vi "32-bit Main.vi"() -> ()   [LabVIEW 2017]
uses:
  <vilib>/express/express analysis/Spectral/Block/exnSpectralBlock spectral measurements peak poly.vi
  <vilib>/express/express analysis/Spectral/Block/exnSpectralBlock spectral measurements peak WFM.vi
  <vilib>/express/express analysis/Spectral/XNode/ExpressSpectralMeasurementsBlockNode.xnode
panel:
  out "Error 401007":errorcluster
  out "Waveform Chart 401007":dbl(graph)
  out "Unsigned Byte Array 401007":u8[](array[numeric])
  out "Little Endian":dbl
  in  "Big Endian":dbl
  out "303005":dbl
  out "Error 303005":errorcluster
  out "Error 303005.1":errorcluster
  out "303005.1":dbl
  out "303007":i64
  out "Error 303007":errorcluster
  out "Error 401007":errorcluster
  out "401007":dbl
  out "Error 401001":errorcluster
  out "401001":i64
  out "Error 301001":errorcluster
  out "301001":i64
  out "Error 001001":errorcluster
  out "001001":bool
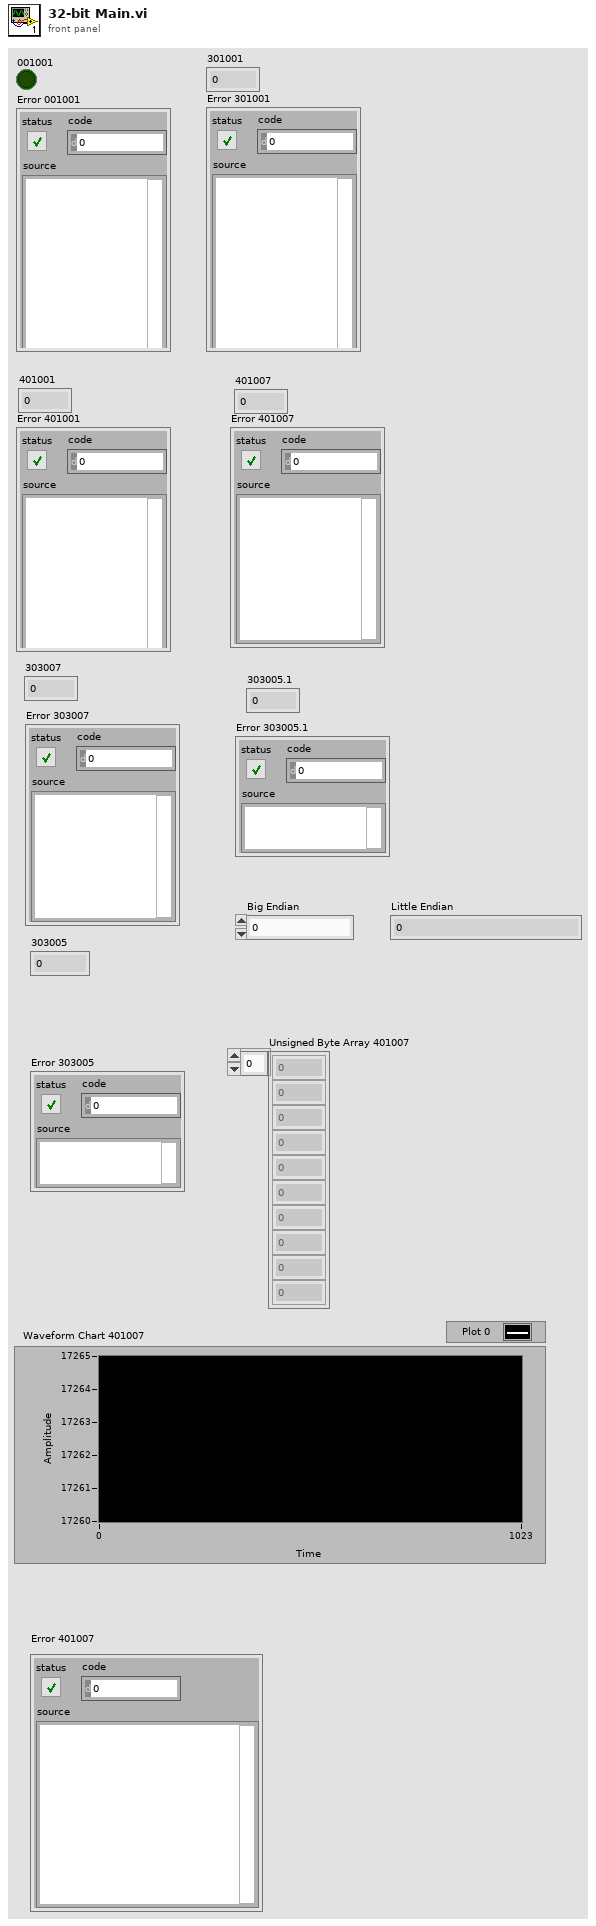
[diagram p1: front panel]
types:
  T1 = enum16{"big-endian, network order", "native, host order", "little-endian"}
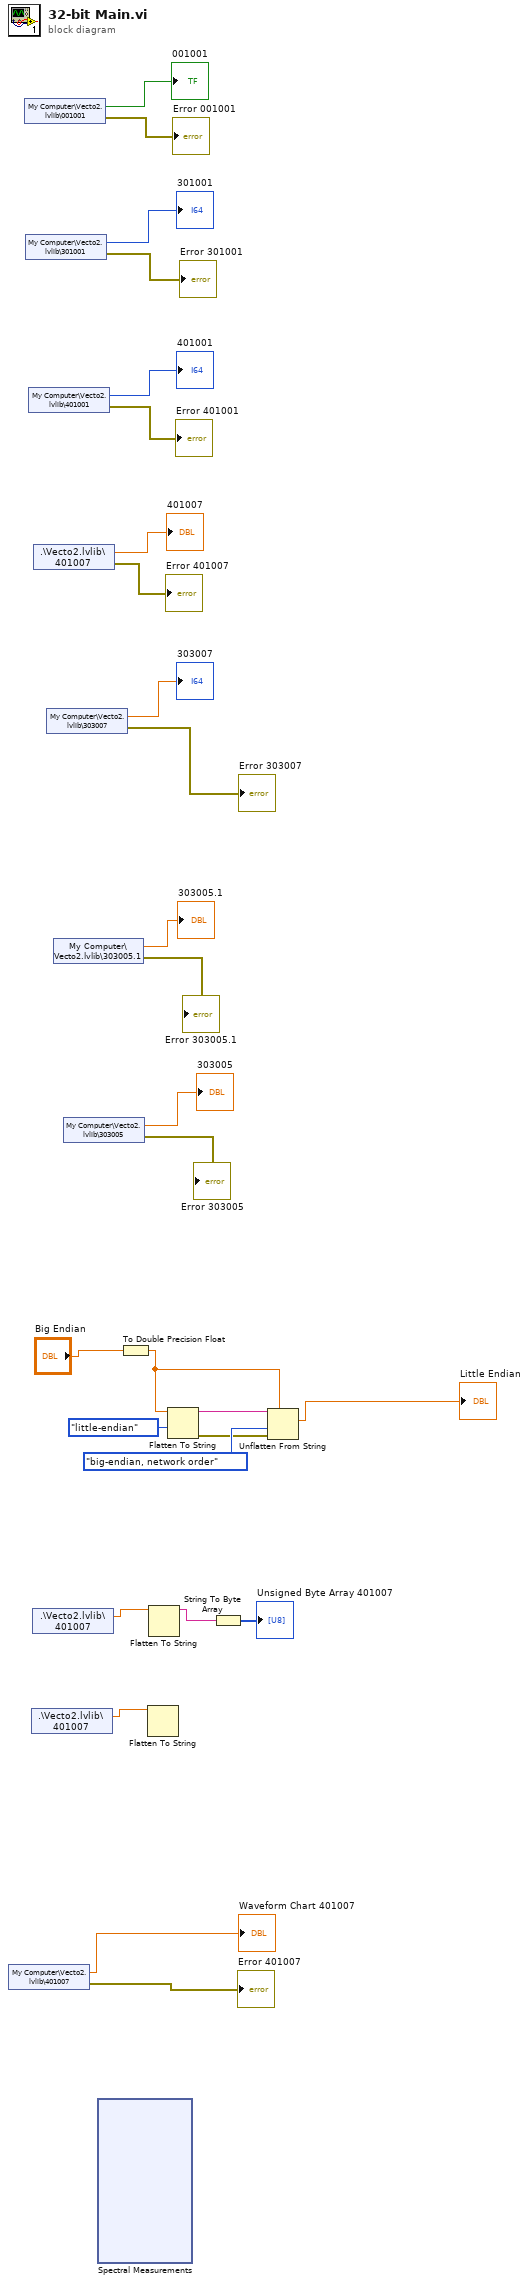
[diagram p0: block diagram]
diagram:
  n1 = shared-variable "My Computer\\Vecto2.lvlib\\401007"() -> (→"Waveform Chart 401007":dbl, error out=→"Error 401007":errorcluster)  [unwired: 1 in]
  n2 = shared-variable "My Computer\\Vecto2.lvlib\\001001"() -> (→"001001":bool, error out=→"Error 001001":errorcluster)  [unwired: 1 in]
  n3 = shared-variable "My Computer\\Vecto2.lvlib\\301001"() -> (→"301001":i64, error out=→"Error 301001":errorcluster)  [unwired: 1 in]
  n4 = shared-variable "My Computer\\Vecto2.lvlib\\401001"() -> (→"401001":i64, error out=→"Error 401001":errorcluster)  [unwired: 1 in]
  n5 = shared-variable ".\\Vecto2.lvlib\\401007"() -> (w2:dbl)  [unwired: 1 in, 1 out]
  n6 = shared-variable ".\\Vecto2.lvlib\\401007"() -> (w7:dbl)  [unwired: 1 in, 1 out]
  n7 = shared-variable ".\\Vecto2.lvlib\\401007"() -> (→"401007":dbl, error out=→"Error 401007":errorcluster)  [unwired: 1 in]
  n8 = shared-variable "My Computer\\Vecto2.lvlib\\303007"() -> (→"303007":sgl, error out=→"Error 303007":errorcluster)  [unwired: 1 in]
  n9 = shared-variable "My Computer\\Vecto2.lvlib\\303005.1"() -> (→"303005.1":dbl, error out=→"Error 303005.1":errorcluster)  [unwired: 1 in]
  n10 = shared-variable "My Computer\\Vecto2.lvlib\\303005"() -> (→"303005":dbl, error out=→"Error 303005":errorcluster)  [unwired: 1 in]
  n11 = xnode "Spectral Measurements"() -> ()  [unwired: 2 in, 3 out]
  n12 = To Double Precision Float(number="Big Endian") -> (double precision float=w9:dbl)
  n13 = Flatten To String(anything=w2) -> ()  [unwired: 3 in, 3 out]
  n14 = Flatten To String(anything=w7) -> (data string=w6:string)  [unwired: 3 in, 2 out]
  n15 = Flatten To String(anything=w9, byte order (0:big-endian, network order)=T1."little-endian") -> (data string=w10:string, error out=w4:errorcluster)  [unwired: 2 in, 1 out]
  n16 = String To Byte Array(string=w6) -> (unsigned byte array=→"Unsigned Byte Array 401007":u8[])
  n17 = Unflatten From String(type=w9, binary string=w10, byte order (0:big-endian, network order)=T1."big-endian, network order", error in (no error)=w4) -> (value=→"Little Endian":dbl)  [unwired: 1 in, 2 out]
